vi "Get CYMG Shift.vi"(10 "iYShift":i32, 11 "iXshift":i32) -> (1 "function return":u32, 2 "iYShift out":i32, 3 "iXshift out":i32)   [LabVIEW 2018, in "Copy of Andor SDK.lvlib"]
doc: "EXPNETTYPE unsigned int WINAPI GetCYMGShift(int * iXshift, int * iYShift);"
uses:
  Copy of Andor SDK.lvlib
  <userlib>/Andor SDK/ATMCD32D.dll
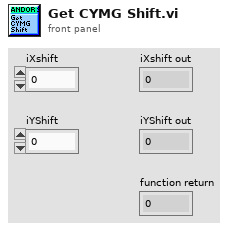
[diagram p1: front panel]
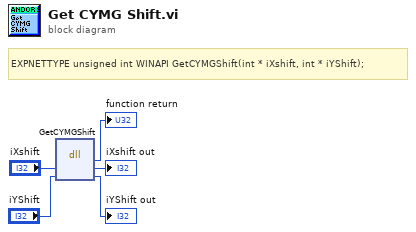
[diagram p0: block diagram]
diagram:
  # "EXPNETTYPE unsigned int WINAPI GetCYMGShift(int * iXshift, int * iYShift);"
  n1 = dll-call lib="C:/Program Files (x86)/National Instruments/LabVIEW 2018/user.lib/Andor SDK/ATMCD32D.*" fn="GetCYMGShift"("iXshift"="iXshift", "iYShift"="iYShift") -> (→"function return":u32, "iXshift"=→"iXshift out":i32, "iYShift"=→"iYShift out":i32)  [unwired: 3 in, 2 out]
